vi "LinearSensorCal.vi"(9 "Sensor Config":cluster{"Sensor Low":dbl, "Sensor Hi":dbl}, 10 "Mech Config":cluster{"Mechanism Hi":dbl, "Mechanism Low":dbl}, 11 "Sense":dbl) -> (3 "Cal Sense":dbl)   [LabVIEW 2017]
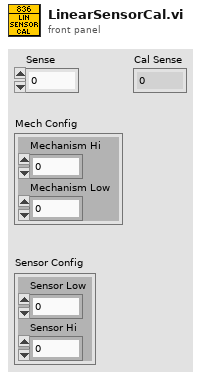
[diagram p1: front panel]
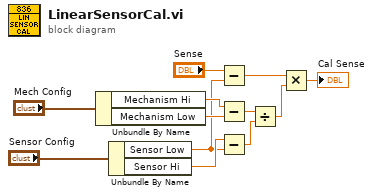
[diagram p0: block diagram]
diagram:
  n1 = Unbundle By Name("Mech Config") -> ("Mechanism Hi"=w9:dbl, "Mechanism Low"=w8:dbl)
  n2 = Unbundle By Name("Sensor Config") -> ("Sensor Low"=w6:dbl, "Sensor Hi"=w7:dbl)
  n3 = Subtract(x="Sense", y=w6) -> (x-y=w2:dbl)
  n4 = Subtract(x=w9, y=w8) -> (x-y=w5:dbl)
  n5 = Subtract(x=w7, y=w6) -> (x-y=w4:dbl)
  n6 = Divide(x=w5, y=w4) -> (x/y=w3:dbl)
  n7 = Multiply(x=w2, y=w3) -> (x*y=→"Cal Sense":dbl)
